vi "aoc-2025-d05-1.vi"() -> ()   [LabVIEW 2025]
uses:
  <vilib>/Utility/error.llb/Trim Whitespace One-Sided.vi
panel:
  out "ans":i32
  out "ingredient ID":u64[](array[numeric])
  out "ranges":u64[][](array[numeric])
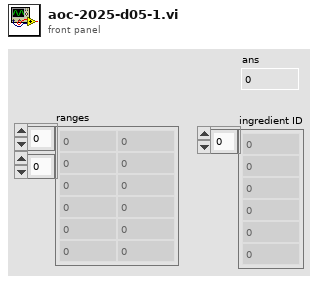
[diagram p1: front panel]
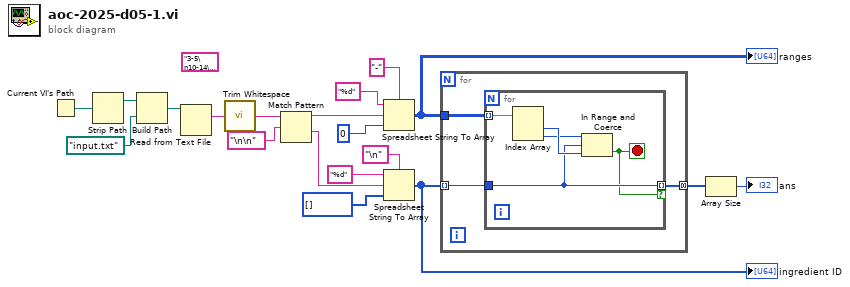
[diagram p0: block diagram]
diagram:
  (unwired) "3-5\n10-14\n16-20\n12-18\n\n1\n5\n8\n11\n17\n32"
  n1 = Current VI's Path() -> (path=w6:path)
  n2 = Strip Path(path=w6) -> (stripped path=w5:path)  [unwired: 1 out]
  n3 = Build Path(base path=w5, name or relative path=path "input.txt") -> (appended path=w3:path)
  n4 = Read from Text File(file (use dialog)=w3) -> (text=w2:string)  [unwired: 3 in, 3 out]
  n5 = call <vilib>:"Trim Whitespace.vi"("string"=w2) -> ("trimmed string"=w1:string)  [unwired: 1 in]
  n6 = Match Pattern(string=w1, regular expression="\n\n") -> (before substring=w18:string, after substring=w14:string)  [unwired: 1 in, 2 out]
  n7 = Spreadsheet String To Array(delimiter (Tab)="-", format string="%d", spreadsheet string=w18, array type (2D Dbl)=u64 0) -> (array=w9:u64[][])
  "ranges" <- w9
  n8 = Spreadsheet String To Array(delimiter (Tab)="\n" ("regular expression"), format string="%d", spreadsheet string=w14, array type (2D Dbl)=u64[] []) -> (array=w10:u64[])
  "ingredient ID" <- w10
  n9 = for {
    tunnel: w10 -> [w22] mode=indexing
    tunnel: w9 -> [w21]
    tunnel: [w20] -> w8 mode=concatenating
    n10 = for {
      tunnel: w22 -> [w24]
      tunnel: w21 -> [w27] mode=indexing
      tunnel: [w24] -> w20 mode=indexing if=w23
      stop <- w23 stop-if-true
      n11 = Index Array(array=w27) -> (element #1=w26:u64, element #2=w25:u64)  [unwired: 2 in]
      n12 = In Range and Coerce(upper limit=w25, x=w24, lower limit=w26) -> (In Range?=w23:bool)  [unwired: 1 out]
    }
  }
  n13 = Array Size(array=w8) -> (size(s)=→"ans":i32)
